vi "GetDisplayName.vi"(8 "error in (no error)":errorcluster, 11 "IRuleFileParser in":refnum<class "IRuleFileParser.lvclass">) -> (0 "error out":errorcluster, 1 "Display name":string, 3 "IRuleFileParser out":refnum<class "IRuleFileParser.lvclass">)   [LabVIEW 2020, in "ExtensionInterfaces.lvlib" / "IRuleFileParser.lvclass"]
uses:
  IRuleFileParser.lvclass
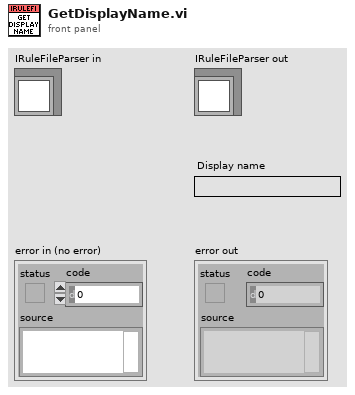
[diagram p1: front panel]
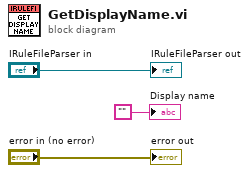
[diagram p0: block diagram]
diagram:
  "error out" <- "error in (no error)"
  "IRuleFileParser out" <- "IRuleFileParser in"
  "Display name" <- ""
